vi "Test.vi"() -> ()   [LabVIEW 2020]
panel:
  out "error out":errorcluster
  out "Execute":bool
  out "data":dbl[](array[numeric])
  out "Table Size":dbl
  in  "Entries":i32
  in  "Start":i32
  out "Table Values":string[][](table)
  out "GetTable":bool
  out "Scope":bool
  out "Trigger 2":bool
  in  "Trigger":bool
  in  "STOP":bool
  in  "Setup Tab":enum32{"SETUP", "MONITORING", "ERRORS"}(tab)
  out "IsOpen":bool
  in  "Connection?":refnum<k7>(container)
  in  "Connect  to Controller":bool=TRUE
  in  "Set Parameters":bool
  in  "Controller Connection Type":string(combo)="2"
  out "Controller Type":string
  out "Product Name":string
  out "Version":string
  out "Serial Port":fxp<+,3,3>
  in  "Save Directory":path
  out "Controller  Error":errorcluster
  out "Laser Sensor Error":errorcluster
  # "CONTROLLER SETTINGS"
  # "LASER DISPLACEMENT SETTINGS"
  # "LINEAR AXIS FEEDBACK"
  # "Current Position \n(mm)"
  # "End Position \n(mm)"
  # "Travel Remaining \n(mm)"
  # "Velocity \n(mm/s2)"
  # "X AXIS"
  # "Encoder"
  # "ROTARY AXIS FEEDBACK"
  # "Current Position \n(deg)"
  # "End Position \n(deg)"
  # "Travel Remaining \n(deg)"
  # "Velocity \n(deg/s2)"
  # "A AXIS"
  # "Encoder"
  # "CONTROLLER"
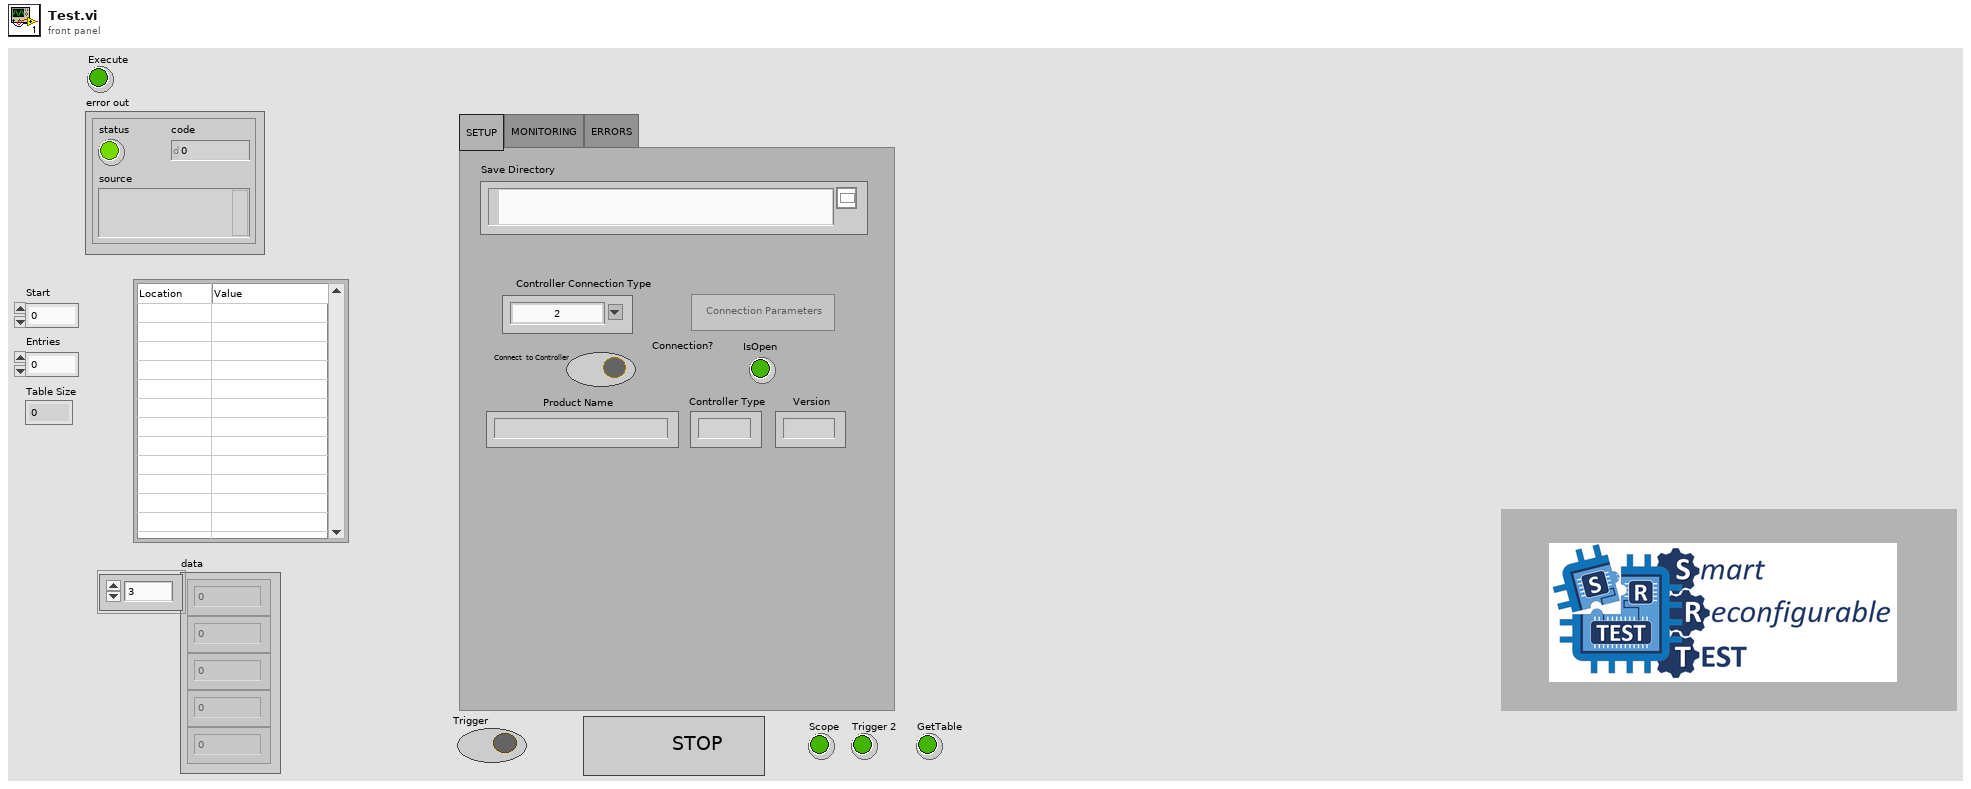
[diagram p1: front panel]
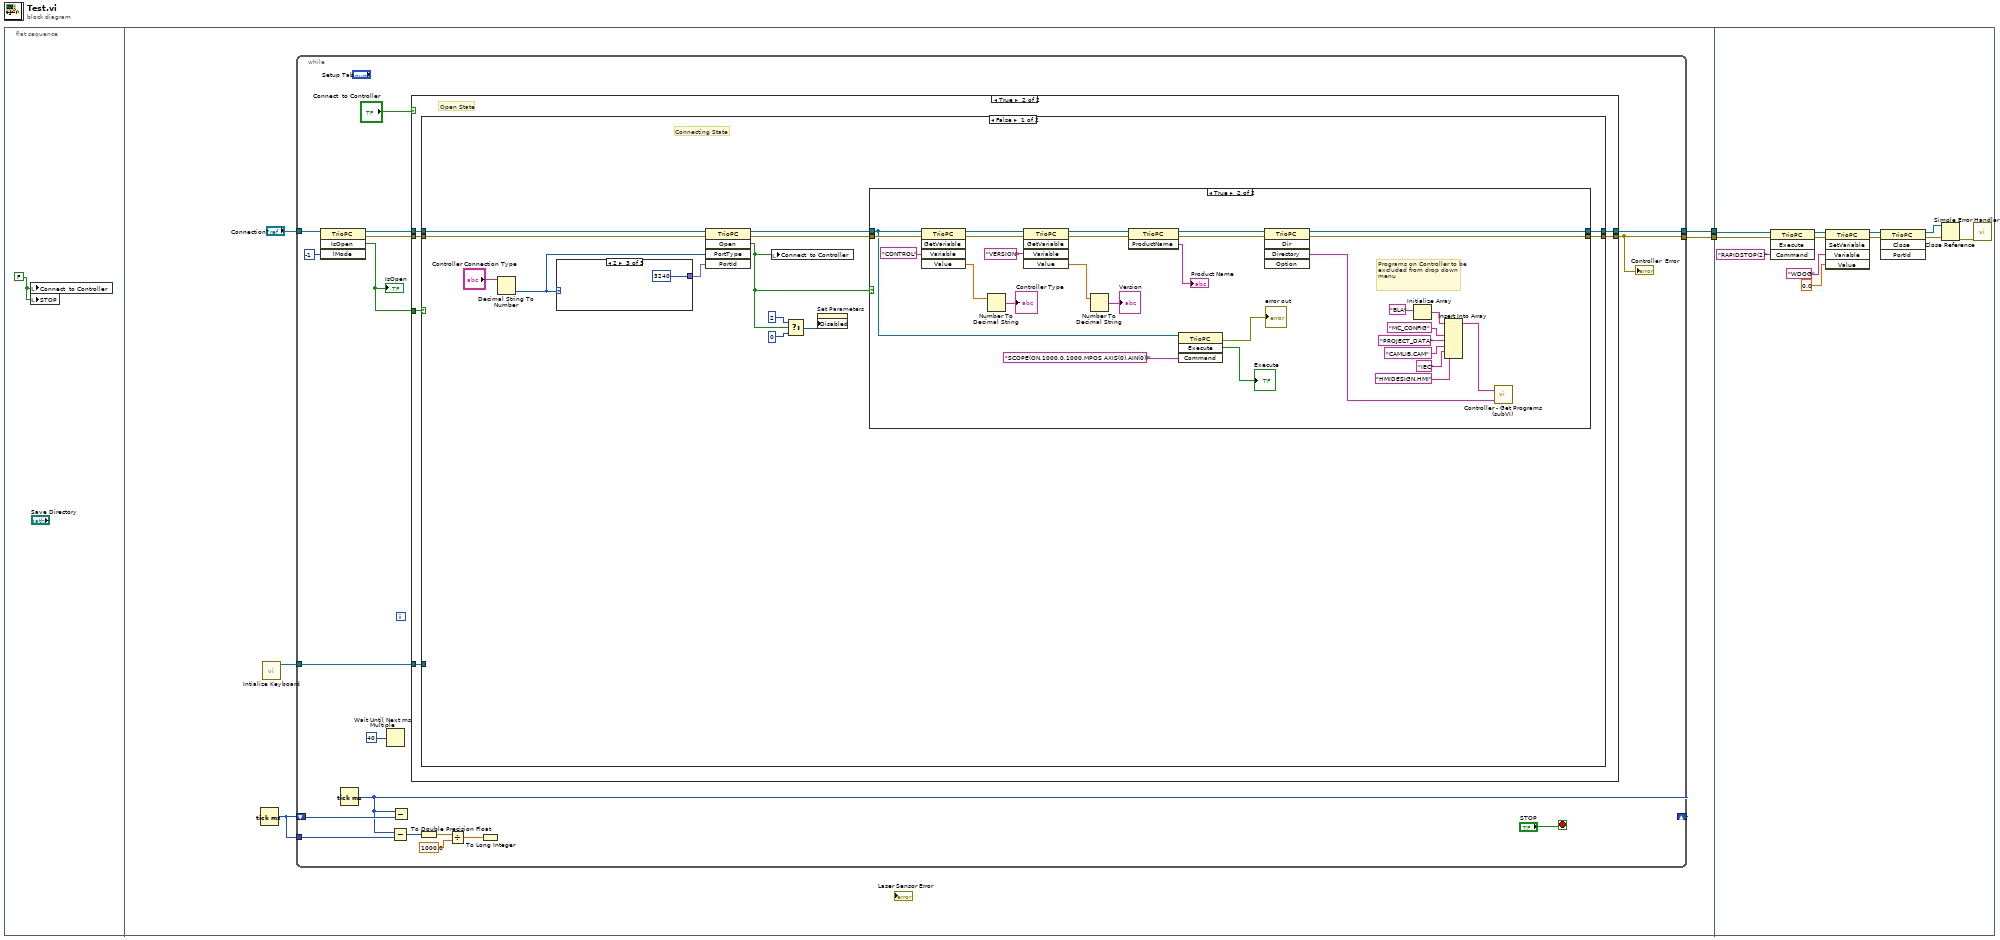
[diagram p0: block diagram]
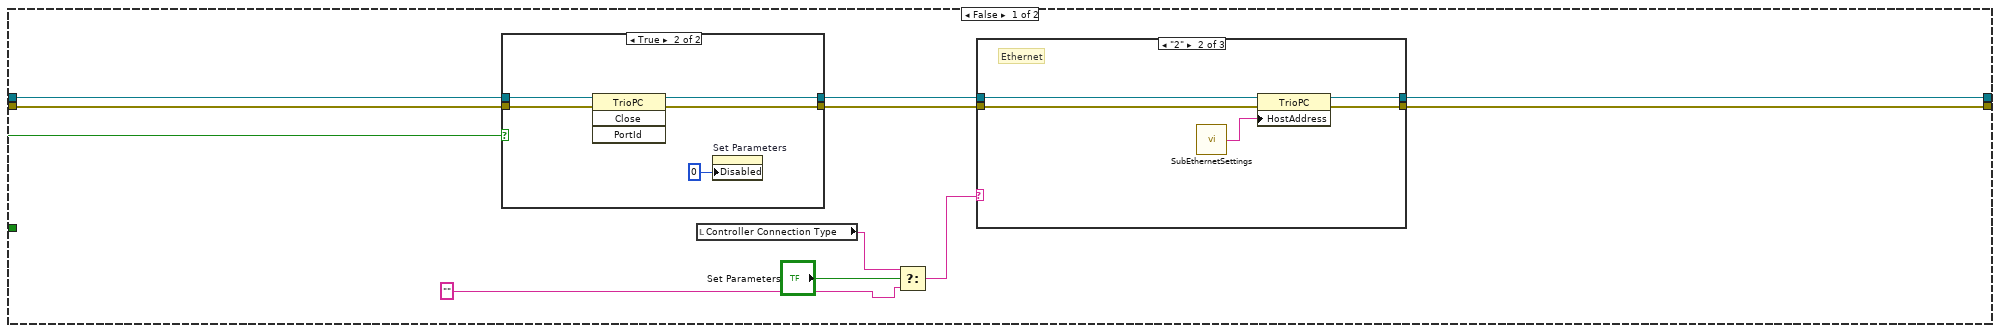
[diagram p2: hidden frame]
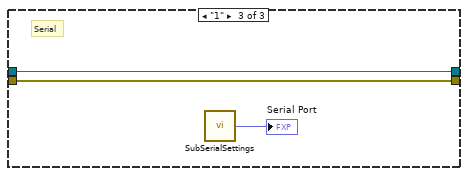
[diagram p5: hidden frame]
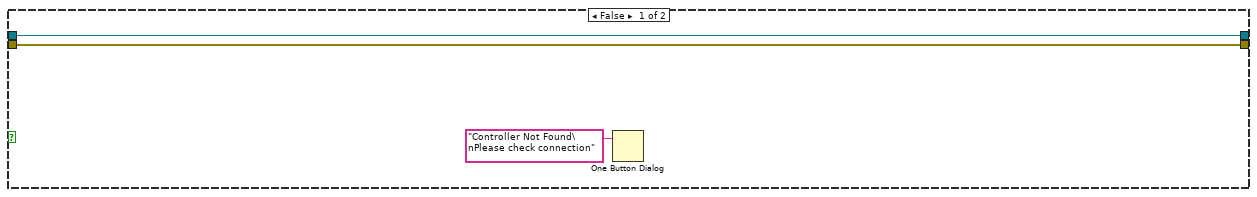
[diagram p6: hidden frame]
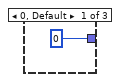
[diagram p7: hidden frame]
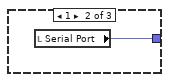
[diagram p8: hidden frame]
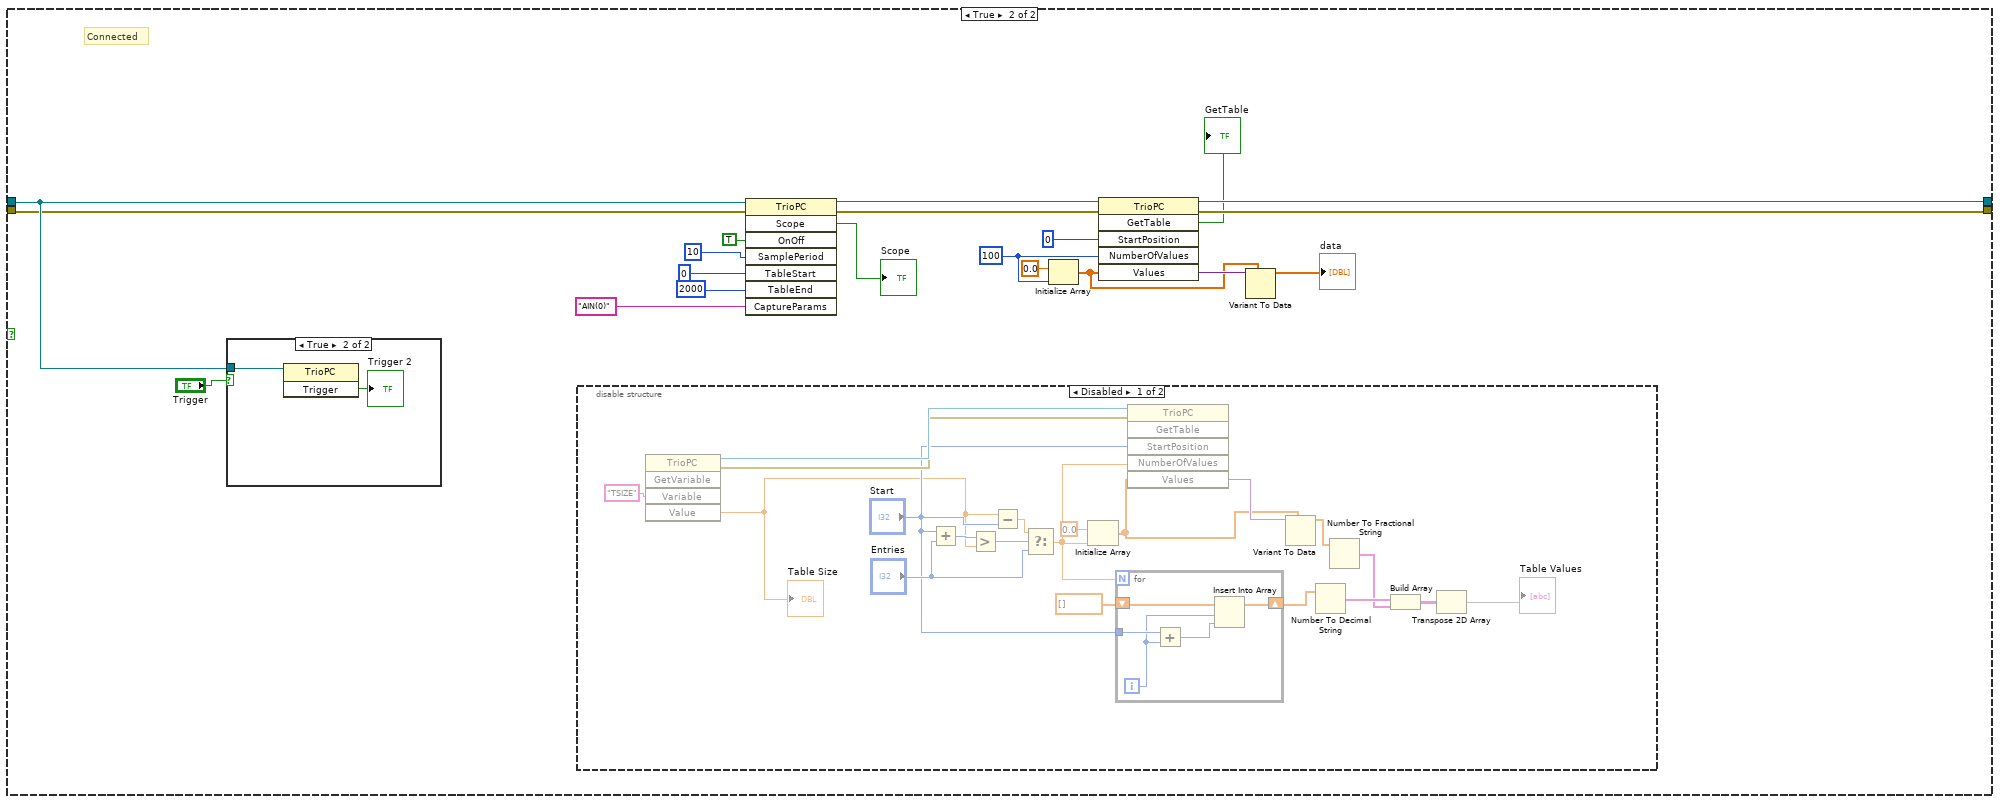
[diagram p9: hidden frame]
diagram:
  n1 = flat-sequence {
    tunnel: [w7] -> w2
    tunnel: [w6] -> w1
    tunnel: w2 -> [w163]
    tunnel: w1 -> [w164]
    frame #0 {
      w3 = FALSE ("Jog Axes")
      n2 = local write "Connect  to Controller"(w3) -> ()
      n3 = local write "STOP"(w3) -> ()
    }
    frame #1 {
      n4 = Tick Count (ms)() -> (millisecond timer value=w5:u32)
      n5 = call <vilib>:"Intialize Keyboard.vi"() -> ("device ID"=w4:refnum<k1>)  [unwired: 1 in, 10 out]
      n6 = while {
        tunnel: "Connection?" -> [w25]
        tunnel: [w22] -> w7
        tunnel: [w13] -> w6
        shift-right: [w16] -> _
        shift-left: w5 -> [w18]
        tunnel: w5 -> [w15]
        tunnel: w4 -> [w12]
        stop <- "STOP" stop-if-true
        n7 = invoke class="TrioPC" method="IsOpen"(reference=w25, "lMode"=-1) -> (reference out=w11:refnum<k7>, error out=w10:errorcluster, "IsOpen"=w23:bool)  [unwired: 2 in, 1 out]
        "IsOpen" <- w23
        n8 = Tick Count (ms)() -> (millisecond timer value=w16:u32)
        n9 = Wait Until Next ms Multiple(millisecond multiple=u32 40) -> ()  [unwired: 1 out]
        n10 = Subtract(x=w16, y=w15) -> (x-y=w14:u32)
        n11 = Subtract(x=w16, y=w18) -> ()  [unwired: 1 out]
        n12 = case shown="True" "Connect  to Controller" {
          tunnel: [w31 w60] -> w22
          tunnel: [w32 w59] -> w13
          tunnel: w23 -> [w28 w58]
          tunnel: w11 -> [w30 w57]
          tunnel: w10 -> [w29 w56]
          tunnel: w12 -> [_ w55]
          frame False {
            n13 = case shown="True" w28 {
              tunnel: [w39 w44] -> w34
              tunnel: [w38 w43] -> w33
              tunnel: w30 -> [w39 w41]
              tunnel: w29 -> [w38 w40]
              frame False {
              }
              frame True {
                n14 = invoke class="TrioPC" method="Close"(reference=w41, error in=w40) -> (reference out=w44:refnum<k7>, error out=w43:errorcluster)  [unwired: 2 in, 2 out]
                n15 = property on="Set Parameters" class="Bool"("Disabled"=u8 0) -> ()  [unwired: 2 in, 2 out]
              }
            }
            n16 = local read "Controller Connection Type"() -> (w27:string)
            n17 = Select(t=w27, s="Set Parameters", f="") -> (s? t:f=w35:string)
            n18 = case shown="\"2\"" w35 {
              tunnel: w34 -> [w46 w49 w54]
              tunnel: w33 -> [w45 w48 w53]
              tunnel: [w46 w51 w54] -> w31
              tunnel: [w45 w50 w53] -> w32
              frame "", Default {
              }
              frame "2" {
                # "Ethernet"
                n19 = call "SubEthernetSettings.vi"() -> ("Ethernet IP Address 2"=w47:string)
                n20 = property class="TrioPC"(reference=w49, error in=w48, "HostAddress"=w47) -> (reference out=w51:refnum<k7>, error out=w50:errorcluster)
              }
              frame "1" {
                # "Serial"
                n21 = call "SubSerialSettings.vi"() -> ("CommPort"=→"Serial Port":fxp<+,3,3>)
              }
            }
          }
          frame True {
            # "Open State"
            n22 = case shown="False" w58 {
              tunnel: [w64 w116] -> w60
              tunnel: [w65 w120] -> w59
              tunnel: w57 -> [w69 w118]
              tunnel: w56 -> [w68 w117]
              tunnel: w55 -> [_ _]
              frame False {
                # "Connecting State"
                n23 = Decimal String To Number(string="Controller Connection Type") -> (number=w66:i32)  [unwired: 2 in, 1 out]
                n24 = case shown="2" w66 {
                  tunnel: [i16 0 ("PortId") w107 i16 3240 ("PortId")] -> w73
                  frame 0, Default {
                  }
                  frame 1 {
                    n25 = local read "Serial Port"() -> (w107:fxp<+,3,3>)
                  }
                  frame 2 {
                  }
                }
                n26 = invoke class="TrioPC" method="Open"(reference=w69, error in=w68, "PortType"=w66, "PortId"=w73) -> (reference out=w63:refnum<k7>, error out=w62:errorcluster, "Open"=w61:bool)  [unwired: 1 in, 2 out]
                n27 = local write "Connect  to Controller"(w61) -> ()
                n28 = Select(t=u8 2, s=w61, f=u8 0 ("Disabled")) -> (s? t:f=w70:u8)
                n29 = property on="Set Parameters" class="Bool"("Disabled"=w70) -> ()  [unwired: 2 in, 2 out]
                n30 = case shown="True" w61 {
                  tunnel: [w75 w104] -> w65
                  tunnel: [w76 w103] -> w64
                  tunnel: w63 -> [w76 w78]
                  tunnel: w62 -> [w75 w86]
                  frame False {
                    n31 = One Button Dialog(message="Controller Not Found\nPlease check connection") -> ()  [unwired: 1 in, 1 out]
                  }
                  frame True {
                    # "Programs on Controller to be excluded from drop down menu"
                    n32 = invoke class="TrioPC" method="GetVariable"(reference=w78, error in=w86, "Variable"="CONTROL") -> (reference out=w88:refnum<k7>, error out=w87:errorcluster, "Value"=w92:dbl)  [unwired: 2 in, 2 out]
                    n33 = Number To Decimal String(number=w92) -> (decimal integer string=→"Controller Type":string)  [unwired: 1 in]
                    n34 = invoke class="TrioPC" method="GetVariable"(reference=w88, error in=w87, "Variable"="VERSION") -> (reference out=w84:refnum<k7>, error out=w85:errorcluster, "Value"=w91:dbl)  [unwired: 2 in, 2 out]
                    n35 = Number To Decimal String(number=w91) -> (decimal integer string=→"Version":string)  [unwired: 1 in]
                    n36 = invoke class="TrioPC" method="ProductName"(reference=w84, error in=w85) -> (reference out=w83:refnum<k7>, error out=w82:errorcluster, "ProductName"=→"Product Name":string)  [unwired: 1 in]
                    n37 = invoke class="TrioPC" method="Execute"(reference=w78, "Command"="SCOPE(ON,1000,0,1000,MPOS AXIS(0),AIN(0))") -> (error out=→"error out":errorcluster, "Execute"=→"Execute":bool)  [unwired: 2 in, 2 out]
                    n38 = invoke class="TrioPC" method="Dir"(reference=w83, error in=w82) -> (reference out=w103:refnum<k7>, error out=w104:errorcluster, "Directory"=w105:string)  [unwired: 3 in, 2 out]
                    n39 = Initialize Array("BLA" ("element")) -> (w102:string[])  [unwired: 1 in]
                    n40 = Insert Into Array(array=w102, new element #1="MC_CONFIG" ("element"), new element #2="PROJECT_DATA" ("element"), new element #3="CAMLIB.CAM" ("element"), new element #4="IEC" ("element"), new element #5="HMIDESIGN.HMI") -> (w95:string[])  [unwired: 1 in]
                    n41 = call "Controller - Get Programs (subVI).vi"("Controller Directory"=w105, "Exclusion List"=w95) -> ()  [unwired: 1 out]
                  }
                }
              }
              frame True {
                w112 = 100 ("PortId")
                # "Connected"
                n42 = case shown="True" "Trigger" {
                  tunnel: w118 -> [_ w154]
                  frame False {
                  }
                  frame True {
                    n43 = invoke class="TrioPC" method="Trigger"(reference=w154) -> ("Trigger"=→"Trigger 2":bool)  [unwired: 2 in, 2 out]
                  }
                }
                n44 = disable-structure shown="Disabled" {
                  frame Disabled {
                    n45 = invoke class="TrioPC" method="GetVariable"("Variable"="TSIZE") -> (reference out=w138:refnum<k7>, error out=w137:errorcluster, "Value"=w129:dbl)  [unwired: 4 in, 2 out]
                    "Table Size" <- w129
                    n46 = Add(x="Start", y="Entries") -> (x+y=w135:i32)
                    n47 = Greater?(x=w135, y=w129) -> (0:w134:bool)
                    n48 = Subtract(x=w129, y="Start") -> (x-y=w130:dbl)
                    n49 = Select(t=w130, s=w134, f="Entries") -> (s? t:f=w132:dbl)
                    n50 = Initialize Array(0.0 ("disabled index (col)"), w132) -> (w144:dbl[])
                    n51 = for {
                      N: w132 -> [_]
                      shift-right: [w152] -> w142
                      shift-left: dbl[] [] -> [w151]
                      tunnel: "Start" -> [w150]
                      i -> [w148]
                      n52 = Add(x=w150, y=w148) -> (x+y=w149:i32)
                      n53 = Insert Into Array(array=w151, index=w148, new element=w149) -> (w152:dbl[])
                    }
                    n54 = invoke class="TrioPC" method="GetTable"(reference=w138, error in=w137, "StartPosition"="Start", "NumberOfValues"=w132, "Values"=w144) -> ("Values"=w146:variant)  [unwired: 1 in, 5 out]
                    n55 = Variant To Data(type=w144, Variant=w146) -> (data=w140:dbl[])  [unwired: 1 in, 1 out]
                    n56 = Number To Decimal String(number=w142) -> (decimal integer string=w141:string[])  [unwired: 1 in]
                    n57 = Number To Fractional String(number=w140) -> (F-format string=w139:string[])  [unwired: 3 in]
                    n58 = Build Array(w141, w139) -> (w143:string[][])
                    n59 = Transpose 2D Array(2D array=w143) -> (transposed array=→"Table Values":string[][])
                  }
                  frame Enabled {
                  }
                }
                n60 = invoke class="TrioPC" method="Scope"(reference=w118, error in=w117, "OnOff"=TRUE, "SamplePeriod"=10 ("x"), "TableStart"=0 ("x"), "TableEnd"=2000 ("x"), "CaptureParams"="AIN(0)") -> (reference out=w119:refnum<k7>, error out=w120:errorcluster, "Scope"=→"Scope":bool)  [unwired: 1 in, 5 out]
                n61 = Initialize Array(0.0 ("disabled index (col)"), w112) -> (w110:dbl[])
                n62 = invoke class="TrioPC" method="GetTable"(reference=w119, "StartPosition"=0 ("PortId"), "NumberOfValues"=w112, "Values"=w110) -> (reference out=w116:refnum<k7>, "GetTable"=→"GetTable":bool, "Values"=w111:variant)  [unwired: 2 in, 3 out]
                n63 = Variant To Data(type=w110, Variant=w111) -> (data=→"data":dbl[])  [unwired: 1 in, 1 out]
              }
            }
          }
        }
        "Controller  Error" <- w13
        n64 = To Double Precision Float(number=w14) -> (double precision float=w17:dbl)
        n65 = Divide(x=w17, y=1000.0) -> (x/y=w20:dbl)
        n66 = To Long Integer(number=w20) -> ()  [unwired: 1 out]
      }
    }
    frame #2 {
      n67 = invoke class="TrioPC" method="Execute"(reference=w163, error in=w164, "Command"="RAPIDSTOP(2)") -> (reference out=w159:refnum<k7>, error out=w160:errorcluster)  [unwired: 1 in, 2 out]
      n68 = invoke class="TrioPC" method="SetVariable"(reference=w159, error in=w160, "Variable"="WDOG", "Value"=0.0) -> (reference out=w158:refnum<k7>, error out=w157:errorcluster)  [unwired: 1 in, 3 out]
      n69 = invoke class="TrioPC" method="Close"(reference=w158, error in=w157) -> (reference out=w165:refnum<k7>, error out=w166:errorcluster)  [unwired: 2 in, 2 out]
      n70 = Close Reference(reference=w165, error in (no error)=w166) -> (error out=w162:errorcluster)
      n71 = call <vilib>:"Simple Error Handler.vi"("error in (no error)"=w162) -> ()  [unwired: 4 in, 5 out]
    }
  }
